vi "Simple TCP - Client_Modified.vi"() -> ()   [LabVIEW 2020]
doc: "Demonstrates how to open a connection to an TCP server, read the data being sent, and display the data on a chart. This VI is designed to stop if the TCP connection is terminated."
panel:
  in  "bytes to read":i32=50
  out "data out":string="OK\r\n NORTH ATLANTIC,5330A-10,R11207,132.8.15.13.13"
  in  "Server Closed":string="The server VI closed the connection."
  # "Overview: Demonstrates the use of the TCP functions to connect to a TCP server VI and receive data.\nInstructions:\n1. Ensure Simple TCP - Server.vi is already running.\n2. Run the VI.\n3. Click Stop to stop the VI. Note that if you stop the server VI, this VI will stop automatically."
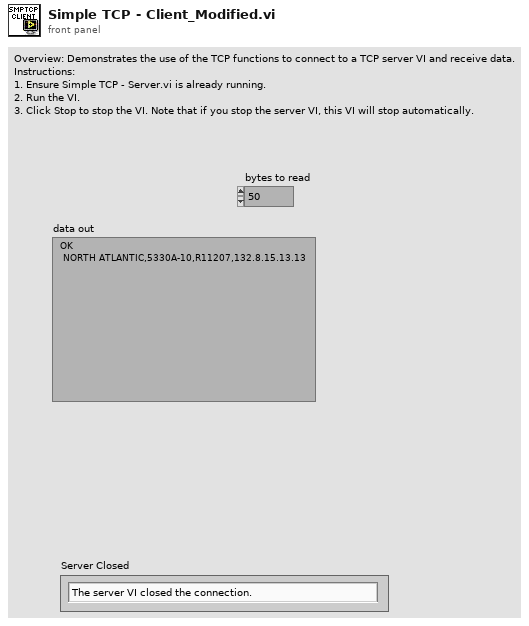
[diagram p1: front panel]
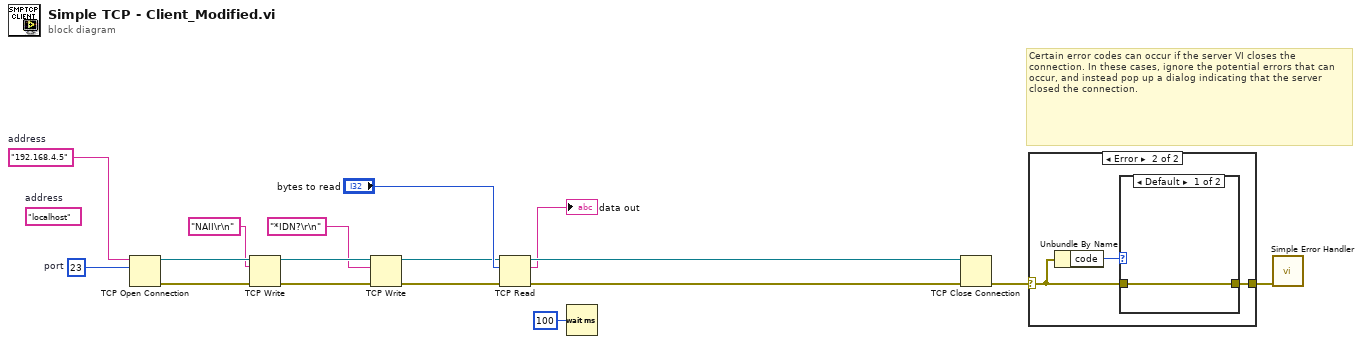
[diagram p0: block diagram]
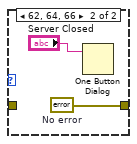
[diagram p3: hidden frame]
diagram:
  w12 = "192.168.4.5"  # address
  w13 = u16 23  # port
  (unwired) "localhost"  # address
  # "Certain error codes can occur if the server VI closes the connection. In these cases, ignore the potential errors that can occur, and instead pop up a dialog indicating that the server closed the connection."
  n1 = TCP Open Connection(address=w12, remote port or service name=w13) -> (connection ID=w17:refnum<k5>, error out=w16:errorcluster)  [unwired: 3 in]
  n2 = TCP Write(connection ID=w17, data in="NAII\r\n", error in (no error)=w16) -> (connection ID out=w4:refnum<k5>, error out=w6:errorcluster)  [unwired: 1 in, 1 out]
  n3 = TCP Write(connection ID=w4, data in="*IDN?\r\n", error in (no error)=w6) -> (connection ID out=w3:refnum<k5>, error out=w5:errorcluster)  [unwired: 1 in, 1 out]
  n4 = TCP Read(connection ID=w3, bytes to read="bytes to read", error in (no error)=w5) -> (connection ID out=w11:refnum<k5>, data out=→"data out":string, error out=w10:errorcluster)  [unwired: 2 in]
  n5 = Wait (ms)(milliseconds to wait=u32 100) -> ()  [unwired: 1 out]
  n6 = TCP Close Connection(connection ID=w11, error in (no error)=w10) -> (error out=w15:errorcluster)  [unwired: 1 in, 1 out]
  n7 = case shown="Error" w15 {
    selector: w15 -> [w18 w20]
    tunnel: [w18 w19] -> w14
    frame No Error {
    }
    frame Error {
      n8 = Unbundle By Name(w20) -> ("code"=w21:i32)
      n9 = case shown="Default" w21 {
        tunnel: w20 -> [w22 _]
        tunnel: [w22 w24] -> w19
        frame Default {
        }
        frame 62, 64, 66 {
          w24 = errorcluster {"status"=FALSE, "code"=0, "source"=""}  # No error
          n10 = One Button Dialog(message="Server Closed") -> ()  [unwired: 1 in, 1 out]
        }
      }
    }
  }
  n11 = call <vilib>:"Simple Error Handler.vi"("error in (no error)"=w14) -> ()  [unwired: 4 in, 5 out]
